vi "周期设置_多参数.vi"() -> ()   [LabVIEW 2016, in "斯坦道多参数.lvlib"]
uses:
  <vilib>/Utility/miscctls.llb/LVPointTypeDef.ctl
  <vilib>/Utility/config.llb/NI_LVConfig.lvlib
panel:
  in  "关闭":bool
  out "执行:状态":T1(ring)
  in  "运行周期":T2
  # "运行模式："
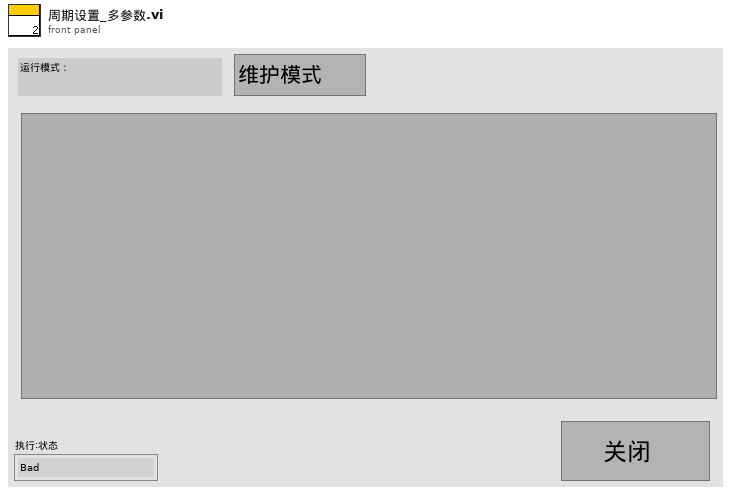
[diagram p1: front panel]
types:
  T1 = enum32{"Bad", "Idle", "Run top level", "Running"}
  T2 = cluster{"运行模式":enum16{"维护模式", "常规模式", "应急模式", "质控模式"}, "24H周期设置":bool[]}
  T3 = typedef "LVPointTypeDef.ctl" = cluster{"Horizontal":i16, "Vertical":i16}
  T4 = typedef "LVDateTimeRec.ctl" = cluster{"秒数的小数部分":dbl, "秒":i32, "分":i32, "时":i32, "日":i32, "月":i32, "年":i32, "天数（周）":i32, "天数（年）":i32, "DST":i32}
  T5 = typedef "NI_LVConfig.lvlib/Config Data RefNum.ctl" = refnum<k1>
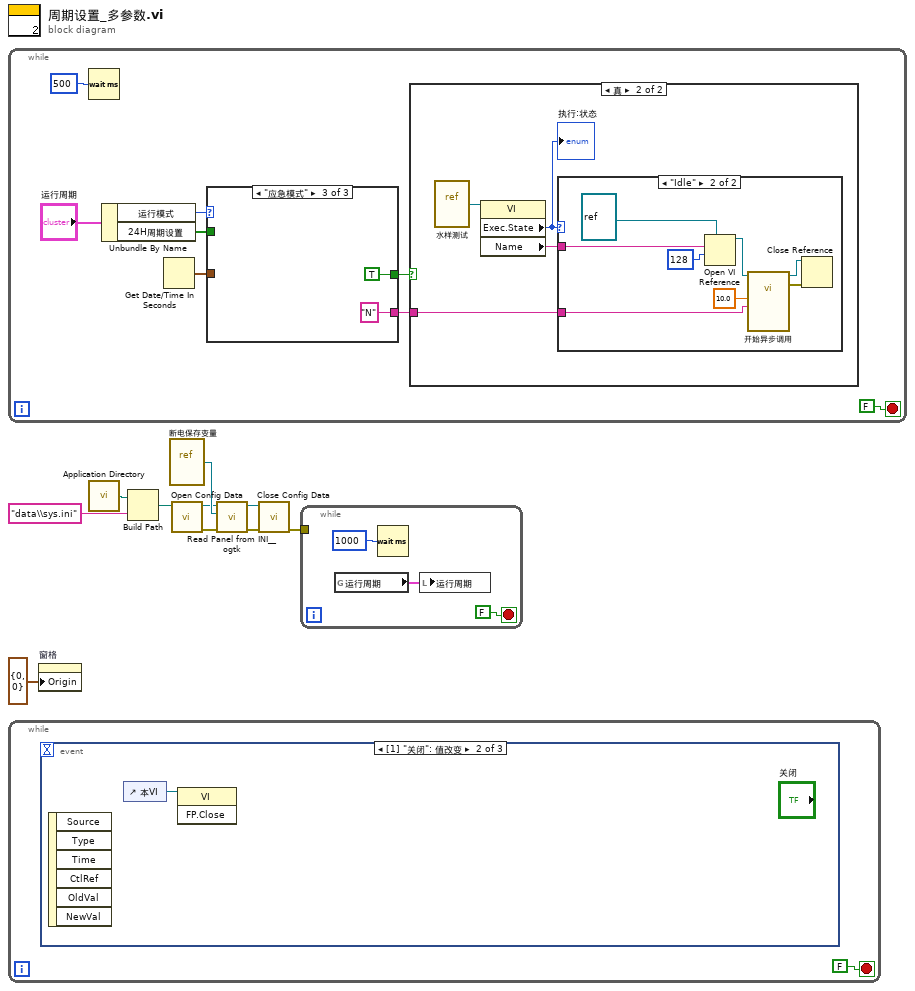
[diagram p0: block diagram]
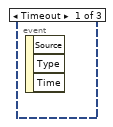
[diagram p2: hidden frame]
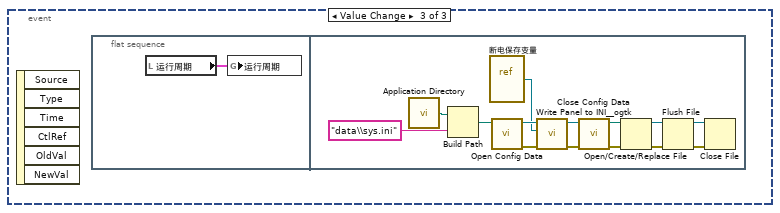
[diagram p3: hidden frame]
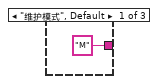
[diagram p6: hidden frame]
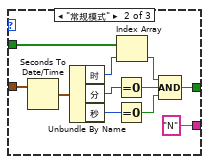
[diagram p7: hidden frame]
diagram:
  n1 = while {
    stop <- FALSE stop-if-true
    n2 = Wait (ms)(milliseconds to wait=u32 500 ("等待时间（毫秒）")) -> ()  [unwired: 1 out]
    n3 = Unbundle By Name("运行周期") -> ("运行模式"=w14:enum16{"维护模式", "常规模式", "应急模式", "质控模式"}, "24H周期设置"=w13:bool[])
    n4 = Get Date/Time In Seconds() -> (seconds since 1Jan1904=w18:timestamp)
    n5 = case shown="\"应急模式\"" w14 {
      tunnel: w18 -> [_ w42 _]
      tunnel: w13 -> [_ w39 _]
      tunnel: [_ w33 TRUE] -> w12
      tunnel: ["M" "N" "N"] -> w11
      frame "维护模式", Default {
      }
      frame "常规模式" {
        n6 = Seconds To Date/Time(time stamp (now)=w42) -> (date time rec=w41:T4)  [unwired: 1 in]
        n7 = Unbundle By Name(w41) -> ("时"=w40:i32, "分"=w38:i32, "秒"=w37:i32)
        n8 = Equal To 0?(x=w38) -> (x = 0?=w35:bool)
        n9 = Equal To 0?(x=w37) -> (x = 0?=w34:bool)
        n10 = Index Array(array=w39, index=w40) -> (element=w36:bool)
        n11 = Compound Arithmetic op=AND ("复合运算")(w36, w35, w34) -> (w33:bool)
      }
      frame "应急模式" {
      }
    }
    n12 = case shown="真" w12 {
      tunnel: w11 -> [_ w19]
      frame False {
      }
      frame True {
        n13 = vi-ref "水样测试.vi"() -> (w21:refnum<vi>)
        n14 = property class="VI"(reference=w21) -> ("Exec.State"=w20:T1, "Name"=w22:string)  [unwired: 1 in, 2 out]
        "执行:状态" <- w20
        n15 = case shown="\"Idle\"" w20 {
          tunnel: w22 -> [_ w27]
          tunnel: w19 -> [_ w24]
          frame "Bad", Default {
          }
          frame "Idle" {
            n16 = Open VI Reference(type specifier VI Refnum (for type only)=refnum<vi> refnum, vi path=w27, options=128 ("选项")) -> (vi reference=w28:refnum<vi>)  [unwired: 3 in, 1 out]
            n17 = call-by-ref "开始异步调用"(reference=w28, "数据标记表"=w24, "水样测试时间"=10.0) -> (reference out=w29:refnum<vi>, error out=w30:errorcluster)  [unwired: 11 in]
            n18 = Close Reference(reference=w29, error in (no error)=w30) -> ()  [unwired: 1 out]
          }
        }
      }
    }
  }
  n19 = while {
    stop <- FALSE stop-if-true
    n20 = event shown="[1] \"关闭\": 值改变" {
      selector: _ -> [_ _ _]
      dyn-events: _ -> [_ _ _]
      timeout: _ -> [_ _ _]
      event Timeout {
        n21 = event-data() -> ()  [unwired: 1 in, 3 out]
      }
      event "关闭": Value Change {
        n22 = event-data() -> ()  [unwired: 1 in, 6 out]
        n23 = control-ref of="本VI"() -> (w46:refnum<vi>)
        n24 = invoke class="VI" method="FP.Close"(reference=w46) -> ()  [unwired: 2 in, 3 out]
      }
      event "运行周期.24H周期设置", "运行周期.运行模式": Value Change {
        n25 = event-data() -> ()  [unwired: 1 in, 6 out]
        n26 = flat-sequence {
          frame #0 {
            n27 = local read "运行周期"() -> (w47:T2)
            n28 = global write "断电保存变量.vi" "运行周期"(w47) -> ()
          }
          frame #1 {
            n29 = call <vilib>:"Application Directory.vi"() -> ("Application Directory"=w61:path)
            n30 = Build Path(base path=w61, name or relative path="data\\sys.ini" ("名称或相对路径")) -> (appended path=w59:path)
            n31 = vi-ref "断电保存变量.vi"() -> (w57:refnum<vi>)
            n32 = call <vilib>:"Open Config Data.vi"("configuration file path"=w59) -> ("error out"=w55:errorcluster, "refnum"=w58:T5)  [unwired: 8 in, 1 out]
            n33 = call <userlib>:"Write Panel to INI__ogtk.vi"("error in (no error)"=w55, "VI ref"=w57, "refnum"=w58) -> ("error out"=w54:errorcluster, "refnum out"=w56:T5)  [unwired: 7 in]
            n34 = call <vilib>:"Close Config Data.vi"("error in (no error)"=w54, "refnum"=w56) -> ("error out"=w49:errorcluster, "file path"=w48:path)  [unwired: 8 in]
            n35 = Open/Create/Replace File(file path (use dialog)=w48, error in=w49) -> (refnum out=w52:refnum<file>, error out=w53:errorcluster)  [unwired: 4 in, 1 out]
            n36 = Flush File(refnum=w52, error in=w53) -> (refnum out=w51:refnum<file>, error out=w50:errorcluster)
            n37 = Close File(refnum=w51, error in=w50) -> ()  [unwired: 2 out]
          }
        }
      }
    }
  }
  n38 = property on="窗格" class="Pane"("Origin"=T3 {"Horizontal"=0, "Vertical"=0} ("原点")) -> ()  [unwired: 2 in, 2 out]
  n39 = call <vilib>:"Application Directory.vi"() -> ("Application Directory"=w3:path)
  n40 = Build Path(base path=w3, name or relative path="data\\sys.ini" ("名称或相对路径")) -> (appended path=w5:path)
  n41 = vi-ref "断电保存变量.vi"() -> (w7:refnum<vi>)
  n42 = call <vilib>:"Open Config Data.vi"("configuration file path"=w5) -> ("error out"=w9:errorcluster, "refnum"=w6:T5)  [unwired: 8 in, 1 out]
  n43 = call <userlib>:"Read Panel from INI__ogtk.vi"("error in (no error)"=w9, "VI ref"=w7, "refnum"=w6) -> ("error out"=w10:errorcluster, "refnum out"=w8:T5)  [unwired: 7 in]
  n44 = call <vilib>:"Close Config Data.vi"("error in (no error)"=w10, "refnum"=w8) -> ("error out"=w2:errorcluster)  [unwired: 8 in, 1 out]
  n45 = while {
    tunnel: w2 -> [_]
    stop <- FALSE stop-if-true
    n46 = global read "断电保存变量.vi" "运行周期"() -> (w62:T2)
    n47 = Wait (ms)(milliseconds to wait=u32 1000 ("等待时间（毫秒）")) -> ()  [unwired: 1 out]
    n48 = local write "运行周期"(w62) -> ()
  }
